vi "Throw Error - Queue Already Exists.vi"(8 "error in (no error)":errorcluster, 11 "Queue Name":string) -> (0 "error out":errorcluster)   [LabVIEW 2022 SP3]
doc: "Issues a command to the Process module by enqueuing into the Process module queue."
panel:
  # "Development\ncontrols/indicators useful for development and testing, but which are not outputs of the VI"
  # "Input\nInputs to the VI"
  # "Output\nOutputs of the VI"
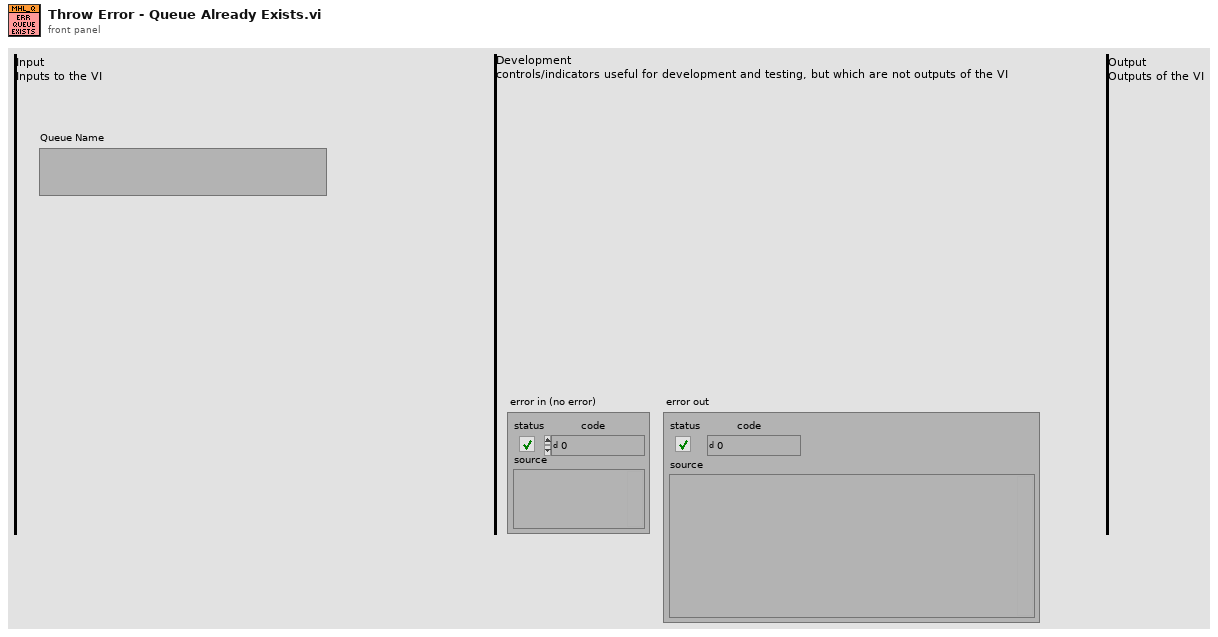
[diagram p1: front panel]
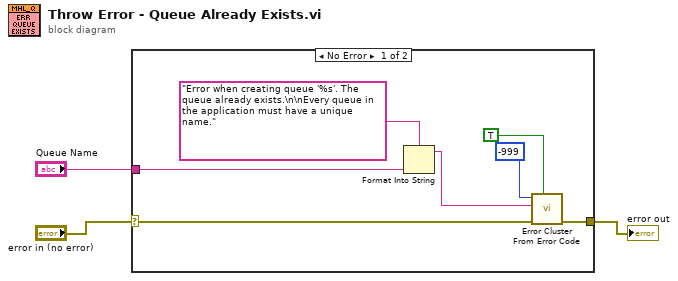
[diagram p0: block diagram]
diagram:
  n1 = case shown="No Error" "error in (no error)" {
    selector: "error in (no error)" -> [w10 w11]
    tunnel: [w9 w11] -> w2
    tunnel: "Queue Name" -> [w4 _]
    frame No Error {
      n2 = Format Into String(format string="Error when creating queue '%s'. The queue already exists.\n\nEvery queue in the application must have a unique name.", w4) -> (resulting string=w7:string)  [unwired: 2 in, 1 out]
      n3 = call <vilib>:"Error Cluster From Error Code.vi"("show call chain? (False)"=TRUE, "error in (no error)"=w10, "error message (\"\")"=w7, "error code (0)"=-999) -> ("error out"=w9:errorcluster)  [unwired: 5 in]
    }
    frame Error {
      # "If error at input, do not overwrite."
    }
  }
  "error out" <- w2
